vi "Write to File.vi"(8 "error in":errorcluster, 10 "DataIn":string, 11 "File in":refnum<class "File.lvclass">) -> (0 "error out":errorcluster, 3 "File out":refnum<class "File.lvclass">)   [LabVIEW 2013, in "File.lvclass"]
uses:
  File.lvclass
  File.lvclass/File.ctl
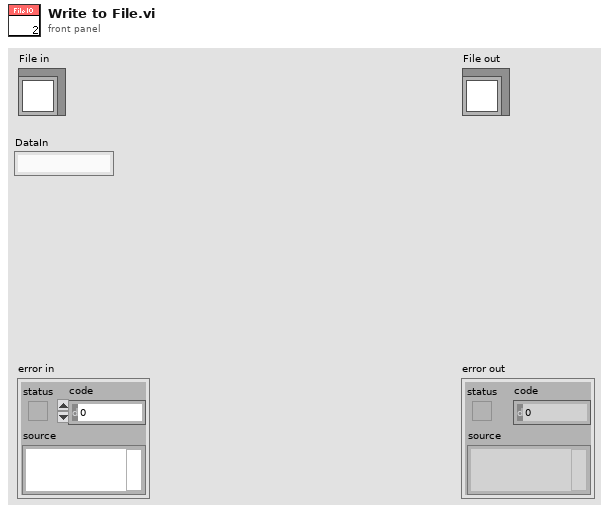
[diagram p1: front panel]
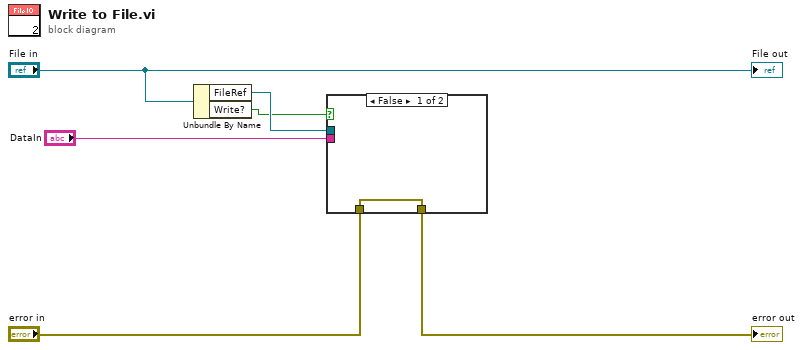
[diagram p0: block diagram]
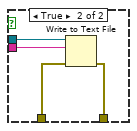
[diagram p2: hidden frame]
diagram:
  n1 = Unbundle By Name("File in") -> ("FileRef"=w5:refnum<file>, "Write?"=w1:bool)
  n2 = case shown="False" w1 {
    tunnel: w5 -> [_ w11]
    tunnel: "error in" -> [w7 w10]
    tunnel: [w7 w9] -> w3
    tunnel: "DataIn" -> [_ w8]
    frame False {
    }
    frame True {
      n3 = Write to Text File(file (use dialog)=w11, text=w8, error in=w10) -> (error out=w9:errorcluster)  [unwired: 1 in, 2 out]
    }
  }
  "error out" <- w3
  "File out" <- "File in"
